vi "Test SPIM7_Keypad API.vi"() -> ()   [LabVIEW 2018]
doc: "SPIM7_Keypad API Tester."
uses:
  SPIM7_Keypad.lvlib
panel:
  out "PelcoD frame":string
  in  "Scan keypad Command":bool
  in  "Close COM port":bool
  in  "Open COM port":bool
  in  "VISA resource name":refnum<visa-resource-name>
  in  "Show Block Diagram":bool
  in  "Stop Module":bool
  in  "Start Module":bool
  in  "Hide Module Panel":bool
  in  "Show Module Panel":bool
  out "Status":string
  out "Module Running?":bool
  # "This VI tests the API for the Module."
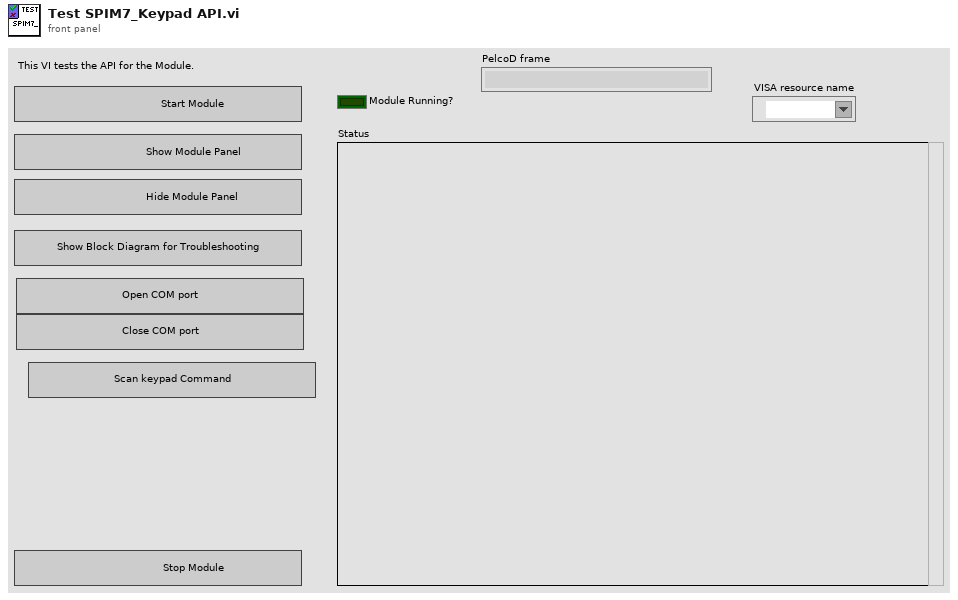
[diagram p1: front panel]
types:
  T1 = typedef "SPIM7_Keypad.lvlib/Broadcast Events--cluster.ctl" = cluster{"Module Did Init":refnum<user-event>, "Status Updated":refnum<user-event>, "Error Reported":refnum<user-event>, "Module Did Stop":refnum<user-event>, "Update Module Execution Status":refnum<user-event>}
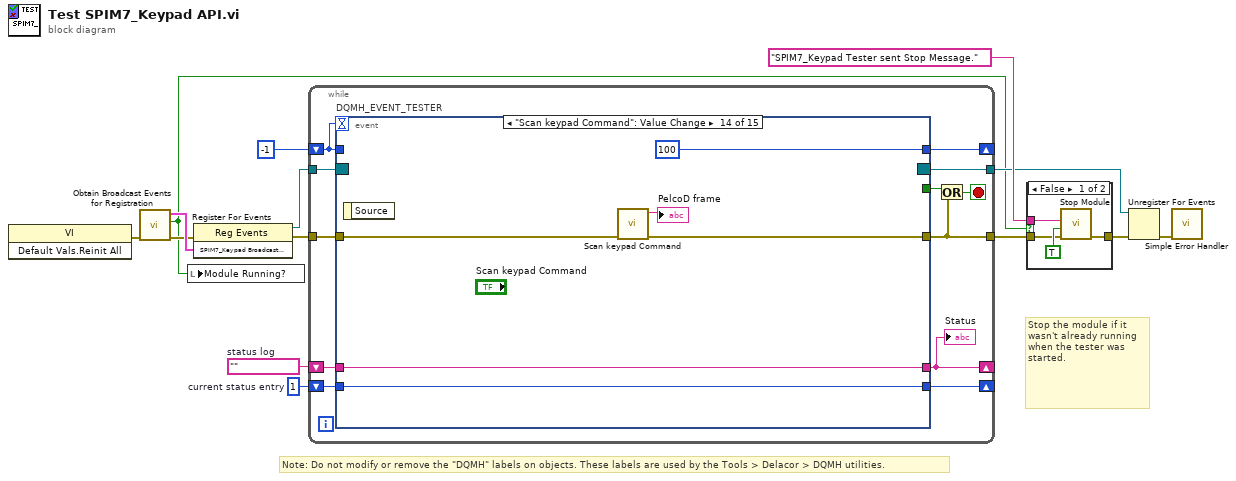
[diagram p0: block diagram]
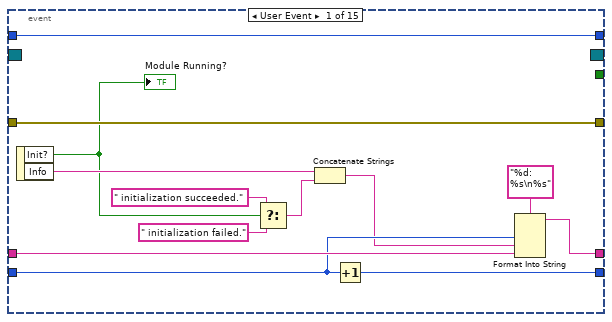
[diagram p3: hidden frame]
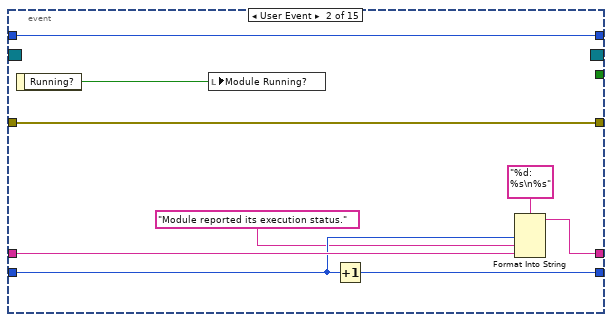
[diagram p4: hidden frame]
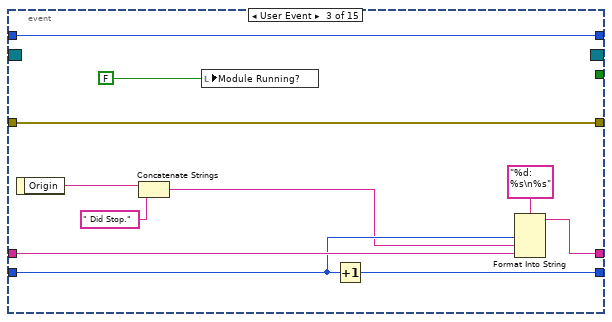
[diagram p5: hidden frame]
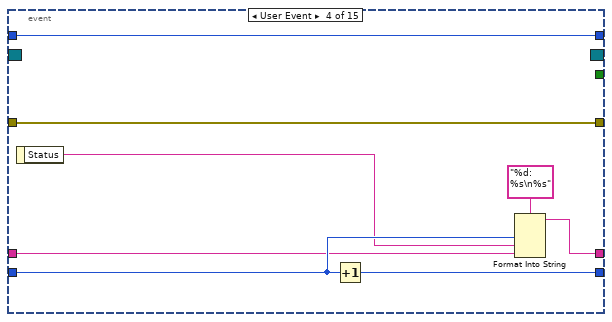
[diagram p6: hidden frame]
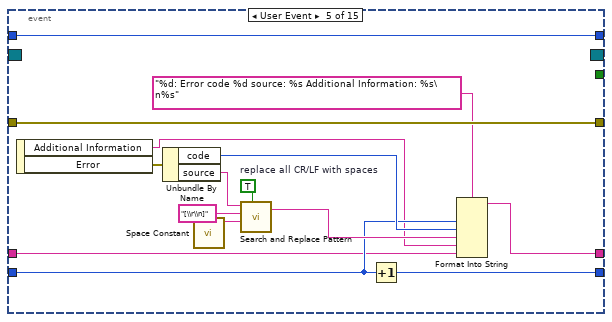
[diagram p7: hidden frame]
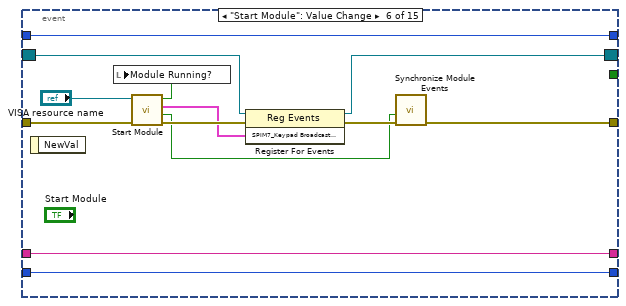
[diagram p8: hidden frame]
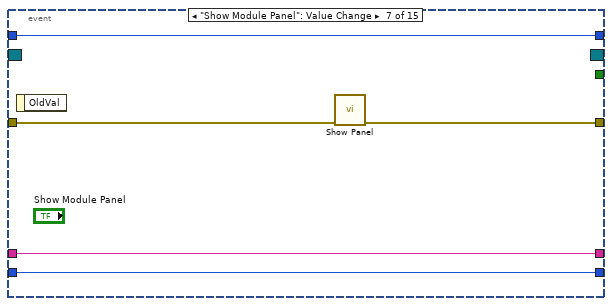
[diagram p9: hidden frame]
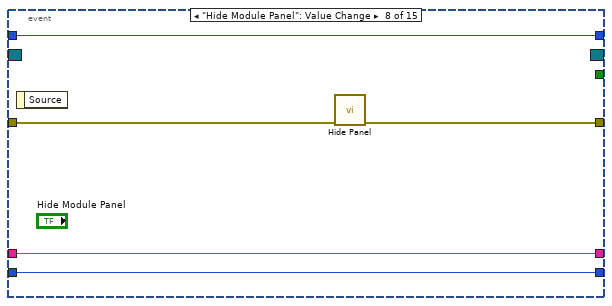
[diagram p10: hidden frame]
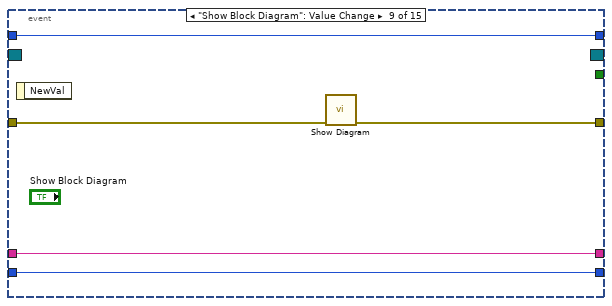
[diagram p11: hidden frame]
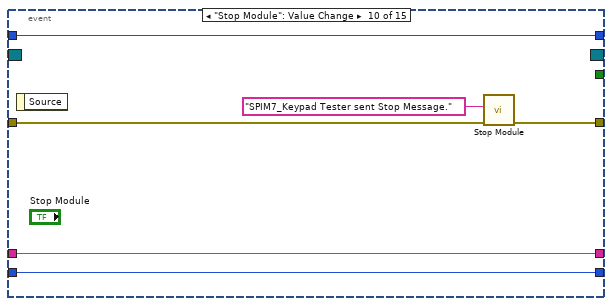
[diagram p12: hidden frame]
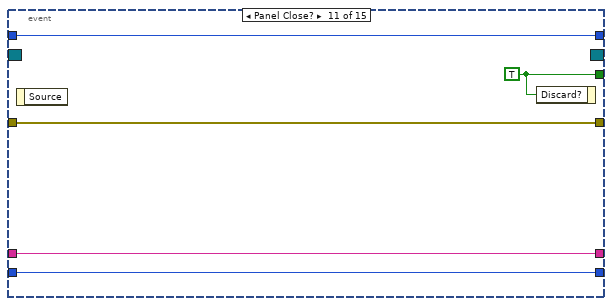
[diagram p13: hidden frame]
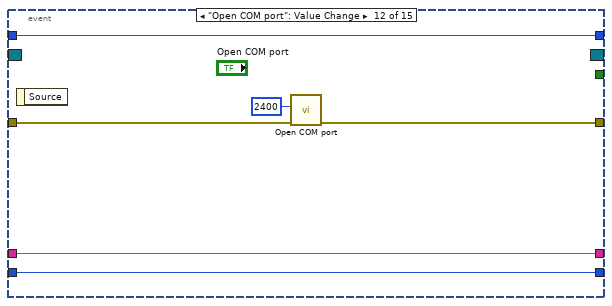
[diagram p14: hidden frame]
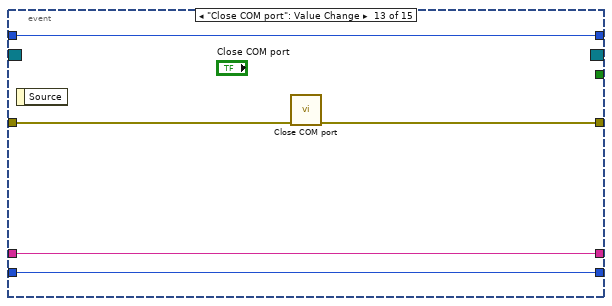
[diagram p15: hidden frame]
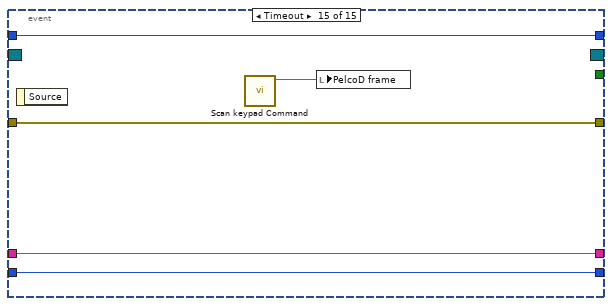
[diagram p16: hidden frame]
diagram:
  w11 = 1  # current status entry
  w12 = ""  # status log
  # "Stop the module if it wasn't already running when the tester was started."
  # "Note: Do not modify or remove the \"DQMH\" labels on objects. These labels are used by the Tools > Delacor > DQMH utilities."
  n1 = invoke class="VI" method="Default Vals.Reinit All"() -> (error out=w6:errorcluster)  [unwired: 3 in, 2 out]
  n2 = call "Obtain Broadcast Events for Registration.vi"("error in (no error)"=w6) -> ("error out"=w5:errorcluster, "Already running?"=w4:bool, "SPIM7_Keypad Broadcast Events"=w9:T1)  [unwired: 8 in]
  n3 = local write "Module Running?"(w4) -> ()
  n4 = register-events(error in=w5, w9) -> (reference out=w8:refnum<event-registration>, error out=w10:errorcluster)  [unwired: 1 in]
  n5 = while {
    tunnel: w8 -> [w26]
    tunnel: [w17] -> w3
    shift-right: [w21] -> _
    shift-left: w12 -> [w23]
    shift-right: [w22] -> _
    shift-left: w11 -> [w24]
    tunnel: w10 -> [w19]
    tunnel: [w18] -> w7
    shift-right: [w16] -> _
    shift-left: -1 -> [w15]
    stop <- w20 stop-if-true
    n6 = event "DQMH_EVENT_TESTER" shown="[13] \"Scan keypad Command\": Value Change" {
      selector: w26 -> [_ _ _ _ _ w89 _ _ _ _ _ _ _ _ _]
      dyn-events: [_ _ _ _ _ w88 _ _ _ _ _ _ _ _ _] -> w18
      timeout: w15 -> [_ _ _ _ _ _ _ _ _ _ _ _ _ _ _]
      tunnel: [_ _ _ _ _ _ _ _ _ _ w121 _ _ _ _] -> w25
      tunnel: [w39 w42 w50 w61 w82 w87 w100 w105 w107 w114 w118 w124 w129 w135 w143] -> w17
      tunnel: w24 -> [w36 w46 w57 w64 w72 w92 w98 w103 w108 w115 w119 w125 w130 w136 w141]
      tunnel: w23 -> [w37 w47 w58 w63 w70 w93 w99 w104 w109 w116 w120 w126 w131 w137 w142]
      tunnel: [w34 w44 w55 w65 w73 w93 w99 w104 w109 w116 w120 w126 w131 w137 w142] -> w21
      tunnel: [w35 w45 w56 w67 w71 w92 w98 w103 w108 w115 w119 w125 w130 w136 w141] -> w22
      tunnel: w19 -> [w39 w42 w50 w61 w82 w86 w97 w102 w110 w112 w118 w127 w132 w138 w143]
      tunnel: [w27 w40 w49 w60 w68 w83 w96 w101 w106 w111 w117 w122 w128 100 w139] -> w16
      tunnel: w15 -> [w27 w40 w49 w60 w68 w83 w96 w101 w106 w111 w117 w122 w128 _ w139]
      event User Event {
        n7 = event-data() -> ("Init?"=w31:bool, "Info"=w33:string)  [unwired: 1 in]
        "Module Running?" <- w31
        n8 = Select(t=" initialization succeeded.", s=w31, f=" initialization failed.") -> (s? t:f=w28:string)
        n9 = Concatenate Strings(w33, w28) -> (w32:string)
        n10 = Increment(x=w36) -> (x+1=w35:i32)
        n11 = Format Into String(format string="%d: %s\n%s", w36, w32, w37) -> (resulting string=w34:string)  [unwired: 2 in, 1 out]
      }
      event User Event {
        n12 = event-data() -> ("Running?"=w41:bool)  [unwired: 1 in]
        n13 = local write "Module Running?"(w41) -> ()
        n14 = Increment(x=w46) -> (x+1=w45:i32)
        n15 = Format Into String(format string="%d: %s\n%s", w46, "Module reported its execution status.", w47) -> (resulting string=w44:string)  [unwired: 2 in, 1 out]
      }
      event User Event {
        n16 = event-data() -> ("Origin"=w54:string)  [unwired: 1 in]
        n17 = Concatenate Strings(w54, " Did Stop.") -> (w53:string)
        n18 = local write "Module Running?"(FALSE ("Module Did Init?")) -> ()
        n19 = Increment(x=w57) -> (x+1=w56:i32)
        n20 = Format Into String(format string="%d: %s\n%s", w57, w53, w58) -> (resulting string=w55:string)  [unwired: 2 in, 1 out]
      }
      event User Event {
        n21 = event-data() -> ("Status"=w62:string)  [unwired: 1 in]
        n22 = Increment(x=w64) -> (x+1=w67:i32)
        n23 = Format Into String(format string="%d: %s\n%s", w64, w62, w63) -> (resulting string=w65:string)  [unwired: 2 in, 1 out]
      }
      event User Event {
        w78 = TRUE  # replace all CR/LF with spaces
        n24 = event-data() -> ("Additional Information"=w69:string, "Error"=w74:errorcluster)  [unwired: 1 in]
        n25 = Unbundle By Name(w74) -> ("code"=w75:i32, "source"=w76:string)
        n26 = call <vilib>:"Space Constant.vi"() -> ("String"=w79:string)
        n27 = call <vilib>:"Search and Replace Pattern.vi"("string"=w76, "regular expression (\"\")"="[\\r\\n]" ("regular expression (\"\")"), "replace string (\"\")"=w79, "replace all? (F)"=w78) -> ("result string"=w77:string)  [unwired: 1 in, 1 out]
        n28 = Increment(x=w72) -> (x+1=w71:i32)
        n29 = Format Into String(format string="%d: Error code %d source: %s Additional Information: %s\n%s", w72, w75, w77, w69, w70) -> (resulting string=w73:string)  [unwired: 2 in, 1 out]
      }
      event "Start Module": Value Change {
        n30 = event-data() -> ()  [unwired: 1 in, 1 out]
        n31 = call "Start Module.vi"("error in (no error)"=w86, "VISA resource name"="VISA resource name") -> ("error out"=w94:errorcluster, "Wait for Event Sync?"=w91:bool, "SPIM7_Keypad Broadcast Events"=w90:T1, "Module Was Already Running?"=w85:bool)  [unwired: 6 in]
        n32 = local write "Module Running?"(w85) -> ()
        n33 = register-events(reference=w89, error in=w94, w90) -> (reference out=w88:refnum<event-registration>, error out=w95:errorcluster)
        n34 = call "Synchronize Module Events.vi"("error in"=w95, "Wait for Event Sync?"=w91) -> ("error out"=w87:errorcluster)  [unwired: 9 in]
      }
      event "Show Module Panel": Value Change {
        n35 = event-data() -> ()  [unwired: 1 in, 1 out]
        n36 = call "Show Panel.vi"("error in (no error)"=w97) -> ("error out"=w100:errorcluster)  [unwired: 10 in]
      }
      event "Hide Module Panel": Value Change {
        n37 = event-data() -> ()  [unwired: 1 in, 1 out]
        n38 = call "Hide Panel.vi"("error in (no error)"=w102) -> ("error out"=w105:errorcluster)  [unwired: 10 in]
      }
      event "Show Block Diagram": Value Change {
        n39 = event-data() -> ()  [unwired: 1 in, 1 out]
        n40 = call "Show Diagram.vi"("error in (no error)"=w110) -> ("error out"=w107:errorcluster)  [unwired: 10 in]
      }
      event "Stop Module": Value Change {
        n41 = event-data() -> ()  [unwired: 1 in, 1 out]
        n42 = call "Stop Module.vi"("error in"=w112, "Origin"="SPIM7_Keypad Tester sent Stop Message.") -> ("error out"=w114:errorcluster)  [unwired: 9 in]
      }
      event Panel Close? {
        w121 = TRUE ("Discard?")
        n43 = event-data() -> ()  [unwired: 1 in, 1 out]
        n44 = event-data("Discard?"=w121) -> ()  [unwired: 1 in, 1 out]
      }
      event "Open COM port": Value Change {
        n45 = event-data() -> ()  [unwired: 1 in, 1 out]
        n46 = call "Open COM port.vi"("error in"=w127, "baudrate"=u32 2400) -> ("error out"=w124:errorcluster)  [unwired: 9 in]
      }
      event "Close COM port": Value Change {
        n47 = event-data() -> ()  [unwired: 1 in, 1 out]
        n48 = call "Close COM port.vi"("error in"=w132) -> ("error out"=w129:errorcluster)  [unwired: 10 in]
      }
      event "Scan keypad Command": Value Change {
        n49 = event-data() -> ()  [unwired: 1 in, 1 out]
        n50 = call "Scan keypad Command.vi"("error in"=w138) -> ("error out"=w135:errorcluster, "PelcoD frame"=→"PelcoD frame":string)  [unwired: 8 in, 1 out]
      }
      event Timeout {
        n51 = event-data() -> ()  [unwired: 1 in, 1 out]
        n52 = call "Scan keypad Command.vi"() -> ("PelcoD frame"=w140:string)  [unwired: 9 in, 2 out]
        n53 = local write "PelcoD frame"(w140) -> ()
      }
    }
    "Status" <- w21
    n54 = Or(x=w25, y=w17) -> (x .or. y?=w20:bool)
  }
  n55 = case shown="False" w4 {
    tunnel: [w147 w148] -> w14
    tunnel: "SPIM7_Keypad Tester sent Stop Message." ("Origin") -> [w146 _]
    tunnel: w3 -> [w144 w148]
    frame False {
      n56 = call "Stop Module.vi"("error in"=w144, "Wait for Module to Stop? (F)"=TRUE ("Wait for Module to stop?"), "Origin"=w146) -> ("error out"=w147:errorcluster)  [unwired: 8 in]
    }
    frame True {
    }
  }
  n57 = Unregister For Events(event registration refnum=w7, error in=w14) -> (error out=w2:errorcluster)
  n58 = call <vilib>:"Simple Error Handler.vi"("error in (no error)"=w2) -> ()  [unwired: 4 in, 5 out]
